vi "nevstop-programming-palette - Post-Install Custom Action.vi"(10 "Variant":variant) -> (0 "error out":errorcluster)   [LabVIEW 2017]
uses:
  <vilib>/Palette API/Palette Menu/Public Type Define/Item.ctl
  <vilib>/Palette API/Palette Menu/Public Type Define/Palette type.ctl
  <vilib>/Palette API/Palette Menu/Palette Menu.lvlib
panel:
  out "concatenated string":string
  out "Array":i32[](array[numeric])
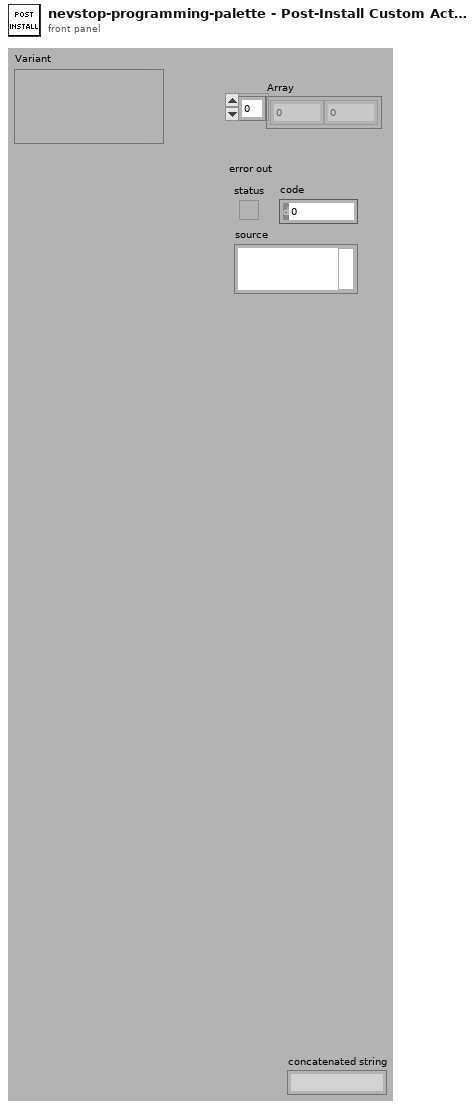
[diagram p1: front panel]
types:
  T1 = typedef "Palette Menu.lvlib/Item.ctl" = cluster{"item path":path, "library path (.lvlib)":path, "use default lvlib palette":bool, "short name":string, "place VI contents":bool, "hide synchronized item":bool, "reserve spot for synch item":bool, "configure when placing VI contents":bool}
  T2 = typedef "Palette Menu.lvlib/Palette type.ctl" = i32
  T3 = typedef "Palette Menu.lvlib/Palette Data.ctl" = cluster{"display name":string, "view format":T4, "palette width":i16, "items":T5, "256 color icon":picture, "B&W color icon":picture, "help information":T6, "palette description":string, "synchronize information":T7}
  T4 = typedef "Palette Menu.lvlib/View Format.ctl" = u16
  T5 = typedef "Palette Menu.lvlib/Items.ctl" = T1[]
  T6 = typedef "Palette Menu.lvlib/Help Info.ctl" = cluster{"help tag":string, "help file path ":path}
  T7 = typedef "Palette Menu.lvlib/Synchronize Info.ctl" = cluster{"synchronize with directory":bool, "synchronize directory path":path}
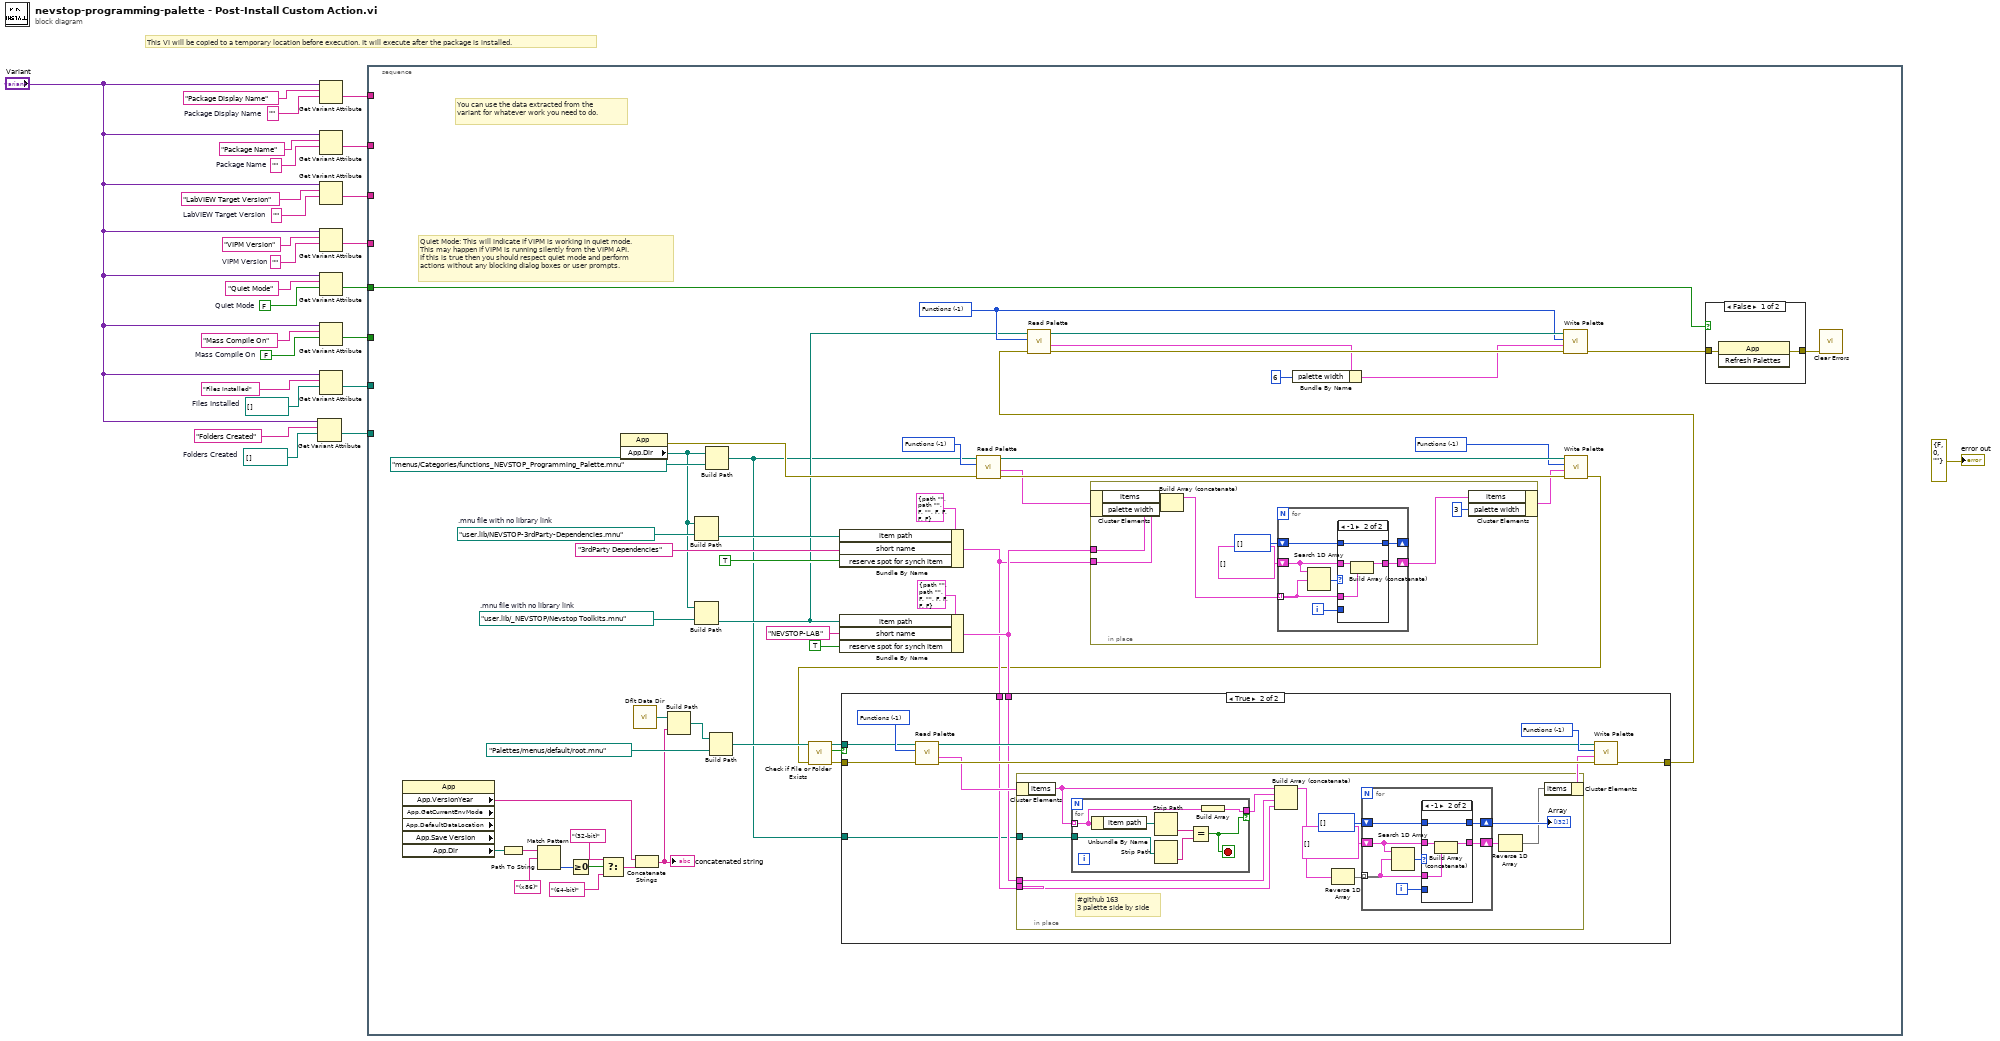
[diagram p0: block diagram]
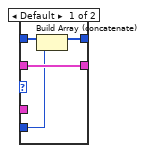
[diagram p3: hidden frame]
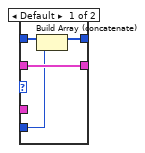
[diagram p4: hidden frame]
diagram:
  w1 = path[] []  # Folders Created
  w2 = path[] []  # Files Installed
  w8 = FALSE  # Mass Compile On
  w9 = ""  # Package Display Name
  w16 = FALSE  # Quiet Mode
  w19 = ""  # VIPM Version
  w21 = ""  # LabVIEW Target Version
  w23 = ""  # Package Name
  # "This VI will be copied to a temporary location before execution. It will execute after the package is installed."
  n1 = Get Variant Attribute(Variant="Variant", name="Folders Created", default value (empty Variant)=w1) -> (value=w6:path[])  [unwired: 1 in, 3 out]
  n2 = Get Variant Attribute(Variant="Variant", name="Package Display Name", default value (empty Variant)=w9) -> (value=w15:string)  [unwired: 1 in, 3 out]
  n3 = Get Variant Attribute(Variant="Variant", name="Package Name", default value (empty Variant)=w23) -> (value=w14:string)  [unwired: 1 in, 3 out]
  n4 = Get Variant Attribute(Variant="Variant", name="LabVIEW Target Version", default value (empty Variant)=w21) -> (value=w13:string)  [unwired: 1 in, 3 out]
  n5 = Get Variant Attribute(Variant="Variant", name="VIPM Version", default value (empty Variant)=w19) -> (value=w12:string)  [unwired: 1 in, 3 out]
  n6 = Get Variant Attribute(Variant="Variant", name="Quiet Mode", default value (empty Variant)=w16) -> (value=w11:bool)  [unwired: 1 in, 3 out]
  n7 = Get Variant Attribute(Variant="Variant", name="Mass Compile On", default value (empty Variant)=w8) -> (value=w10:bool)  [unwired: 1 in, 3 out]
  n8 = Get Variant Attribute(Variant="Variant", name="Files Installed", default value (empty Variant)=w2) -> (value=w5:path[])  [unwired: 1 in, 3 out]
  n9 = stacked-sequence {
    tunnel: w15 -> [_]
    tunnel: w14 -> [_]
    tunnel: w13 -> [_]
    tunnel: w12 -> [_]
    tunnel: w11 -> [w75]
    tunnel: w10 -> [_]
    tunnel: w5 -> [_]
    tunnel: w6 -> [_]
    frame #0 {
      w53 = T2 -1 items=["Functions"=-1, "Controls"=-2] ("palette type")
      w61 = path "user.lib/_NEVSTOP/Nevstop Toolkits.mnu"  # .mnu file with no library link
      w67 = path "user.lib/NEVSTOP-3rdParty-Dependencies.mnu"  # .mnu file with no library link
      w65 = T2 -1 items=["Functions"=-1, "Controls"=-2] ("palette type")
      w63 = T2 -1 items=["Functions"=-1, "Controls"=-2] ("palette type")
      # "Quiet Mode: This will indicate if VIPM is working in quiet mode.\nThis may happen if VIPM is running silently from the VIPM API.\nIf this is true then you should respect quiet mode and perform\nactions without any blocking dialog boxes or user prompts."
      # "You can use the data extracted from the variant for whatever work you need to do."
      n10 = property class="App" props=["App.VersionYear", "App.GetCurrentEnvMode", "App.DefaultDataLocation", "App.Save Version", "App.Dir"]() -> ("App.VersionYear"=w31:string, "App.Dir"=w39:path)  [unwired: 2 in, 5 out]
      n11 = Path To String(path=w39) -> (string=w38:string)
      n12 = Match Pattern(string=w38, regular expression="(x86)") -> (offset past match=w36:i32)  [unwired: 1 in, 3 out]
      n13 = Greater Or Equal To 0?(x=w36) -> (x >= 0?=w35:bool)
      n14 = Select(t="(32-bit)" ("regular expression"), s=w35, f="(64-bit)" ("regular expression")) -> (s? t:f=w32:string)
      n15 = property class="App"() -> (error out=w74:errorcluster, "App.Dir"=w49:path)  [unwired: 2 in, 1 out]
      n16 = call <vilib>:"Dflt Data Dir.vi"() -> ("App:Default Data Directory"=w29:path)
      n17 = Concatenate Strings(w31, w32) -> (w30:string)
      "concatenated string" <- w30
      n18 = Build Path(base path=w29, name or relative path=w30) -> (appended path=w28:path)
      n19 = Build Path(base path=w49, name or relative path=w67) -> (appended path=w73:path)
      n20 = Build Path(base path=w49, name or relative path=w61) -> (appended path=w50:path)
      n21 = Build Path(base path=w49, name or relative path=path "menus/Categories/functions_NEVSTOP_Programming_Palette.mnu") -> (appended path=w27:path)
      n22 = Build Path(base path=w28, name or relative path=path "Palettes/menus/default/root.mnu") -> (appended path=w44:path)
      n23 = Bundle By Name(cluster=T1 {"item path"=path "", "library path (.lvlib)"=path "", "use default lvlib palette"=FALSE, "short name"="", "place VI contents"=FALSE, "hide synchronized item"=FALSE, "reserve spot for synch item"=FALSE, "configure when placing VI contents"=FALSE} ("Items"), "item path"=w73, "short name"="3rdParty Dependencies" ("short name (standard)"), "reserve spot for synch item"=TRUE) -> (w46:T1)
      n24 = Bundle By Name(cluster=T1 {"item path"=path "", "library path (.lvlib)"=path "", "use default lvlib palette"=FALSE, "short name"="", "place VI contents"=FALSE, "hide synchronized item"=FALSE, "reserve spot for synch item"=FALSE, "configure when placing VI contents"=FALSE} ("Items"), "item path"=w50, "short name"="NEVSTOP-LAB" ("short name (standard)"), "reserve spot for synch item"=TRUE) -> (w48:T1)
      n25 = call <vilib>:"Read Palette.vi"("error in (no error)"=w74, "palette type"=w65, "palette path"=w27) -> ("error out"=w71:errorcluster, "palette data"=w62:T3, "duplicate palette path"=w72:path)  [unwired: 1 in, 5 out]
      n26 = in-place {
        in-place-border: w46 -> [w129]
        in-place-border: w48 -> [w130]
        n27 = in-place-cluster #1(w62) -> ("items"=w131:T5)  [unwired: 1 out]
        n28 = Build Array (concatenate)(w131, w130, w129) -> (w125:T5)
        n29 = for {
          tunnel: w125 -> [w137] mode=indexing
          shift-right: [w136] -> w124
          shift-left: T1[] [] -> [w135]
          shift-right: [w133] -> _
          shift-left: i32[] [] -> [w132]
          i -> [w134]
          n30 = Search 1D Array(1D array=w135, element=w137) -> (index of element=w138:i32)  [unwired: 1 in]
          n31 = case shown="-1" w138 {
            tunnel: w137 -> [_ w146]
            tunnel: [w142 w144] -> w136
            tunnel: w135 -> [w142 w145]
            tunnel: w134 -> [w139 _]
            tunnel: [w140 w143] -> w133
            tunnel: w132 -> [w141 w143]
            frame Default {
              n32 = Build Array (concatenate)(w141, w139) -> (w140:i32[])
            }
            frame -1 {
              n33 = Build Array (concatenate)(w145, w146) -> (w144:T1[])
            }
          }
        }
        n34 = in-place-cluster #1("items"=w124, "palette width"=i16 3) -> (w64:T3)
      }
      n35 = call <vilib>:"Write Palette.vi"("error in (no error)"=w71, "palette data"=w64, "palette type"=w63, "palette path"=w72) -> ("error out"=w42:errorcluster)  [unwired: 1 in, 6 out]
      n36 = call <vilib>:"Check if File or Folder Exists.vi"("error in (no error)"=w42, "path"=w44) -> ("error out"=w41:errorcluster, "file or folder exists?"=w40:bool, "dup path"=w43:path)  [unwired: 7 in]
      n37 = case shown="True" w40 {
        tunnel: w48 -> [_ w83]
        tunnel: [w77 w82] -> w47
        tunnel: w46 -> [_ w81]
        tunnel: w43 -> [_ w80]
        tunnel: w41 -> [w77 w79]
        tunnel: w27 -> [_ w78]
        frame False {
        }
        frame True {
          w88 = T2 -1 items=["Functions"=-1, "Controls"=-2] ("palette type")
          w89 = T2 -1 items=["Functions"=-1, "Controls"=-2] ("palette type")
          n38 = call <vilib>:"Read Palette.vi"("error in (no error)"=w79, "palette type"=w88, "palette path"=w80) -> ("error out"=w87:errorcluster, "palette data"=w85:T3, "duplicate palette path"=w86:path)  [unwired: 1 in, 5 out]
          n39 = in-place {
            in-place-border: w83 -> [w101]
            in-place-border: w81 -> [w100]
            in-place-border: w78 -> [w93]
            # "#github 163\n3 palette side by side"
            n40 = in-place-cluster #2(w85) -> ("items"=w94:T5)
            n41 = for {
              tunnel: w94 -> [w104] mode=indexing
              tunnel: w93 -> [w105]
              tunnel: [w103] -> w92 if=w102
              stop <- w102 stop-if-true
              n42 = Unbundle By Name(w104) -> ("item path"=w107:path)
              n43 = Strip Path(path=w107) -> (name=w108:string)  [unwired: 1 out]
              n44 = Strip Path(path=w105) -> (name=w106:string)  [unwired: 1 out]
              n45 = Equal?(x=w108, y=w106) -> (x = y?=w102:bool)
              n46 = Build Array(w104) -> (w103:T1[])
            }
            n47 = Build Array (concatenate)(w94, w92, w101, w100) -> (w99:T5)
            n48 = Reverse 1D Array(array=w99) -> (reversed array=w90:T5)
            n49 = for {
              tunnel: w90 -> [w114] mode=indexing
              shift-right: [w113] -> w96
              shift-left: T1[] [] -> [w112]
              shift-right: [w110] -> w95
              shift-left: i32[] [] -> [w109]
              i -> [w111]
              n50 = Search 1D Array(1D array=w112, element=w114) -> (index of element=w115:i32)  [unwired: 1 in]
              n51 = case shown="-1" w115 {
                tunnel: w114 -> [_ w123]
                tunnel: [w119 w121] -> w113
                tunnel: w112 -> [w119 w122]
                tunnel: w111 -> [w116 _]
                tunnel: [w117 w120] -> w110
                tunnel: w109 -> [w118 w120]
                frame Default {
                  n52 = Build Array (concatenate)(w118, w116) -> (w117:i32[])
                }
                frame -1 {
                  n53 = Build Array (concatenate)(w122, w123) -> (w121:T1[])
                }
              }
            }
            "Array" <- w95
            n54 = Reverse 1D Array(array=w96) -> (reversed array=w91:T1[])
            n55 = in-place-cluster #2("items"=w91) -> (w84:T3)
          }
          n56 = call <vilib>:"Write Palette.vi"("error in (no error)"=w87, "palette data"=w84, "palette type"=w89, "palette path"=w86) -> ("error out"=w82:errorcluster)  [unwired: 1 in, 6 out]
        }
      }
      n57 = call <vilib>:"Read Palette.vi"("error in (no error)"=w47, "palette type"=w53, "palette path"=w50) -> ("error out"=w57:errorcluster, "palette data"=w56:T3, "duplicate palette path"=w54:path)  [unwired: 1 in, 5 out]
      n58 = Bundle By Name(cluster=w56, "palette width"=i16 6) -> (w55:T3)
      n59 = call <vilib>:"Write Palette.vi"("error in (no error)"=w57, "palette data"=w55, "palette type"=w53, "palette path"=w54) -> ("error out"=w51:errorcluster)  [unwired: 1 in, 6 out]
      n60 = case shown="False" w75 {
        tunnel: [w148 w149] -> w76
        tunnel: w51 -> [w147 w149]
        frame False {
          n61 = invoke class="App" method="Refresh Palettes"(error in=w147) -> (error out=w148:errorcluster)  [unwired: 2 in, 2 out]
        }
        frame True {
        }
      }
      n62 = call <vilib>:"Clear Errors.vi"("error in (no error)"=w76) -> ()  [unwired: 5 in, 2 out]
    }
  }
  "error out" <- errorcluster {"status"=FALSE, "code"=0, "source"=""} ("error out")
